vi "update tomo component.vi"(8 "error in (no error)":errorcluster, 11 "Autofocus in":refnum<class "Autofocus.lvclass">) -> (0 "error out":errorcluster, 3 "Autofocus out":refnum<class "Autofocus.lvclass">)   [LabVIEW 2012, in "Autofocus.lvclass"]
uses:
  Autofocus.lvclass
  <vilib>/Distrio/Murmex/Murmex/update_cluster.ctl
  Autofocus.lvclass/Autofocus.ctl
  <vilib>/Distrio/Murmex/Murmex/Murmex.lvclass
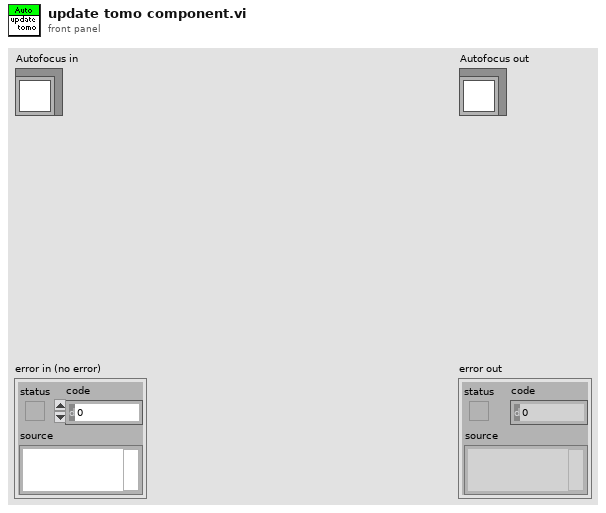
[diagram p1: front panel]
types:
  T1 = typedef "Murmex.lvlib/Murmex.lvclass/update_cluster.ctl" = cluster{"target ID":string, "key chains":string[], "values":variant[]}
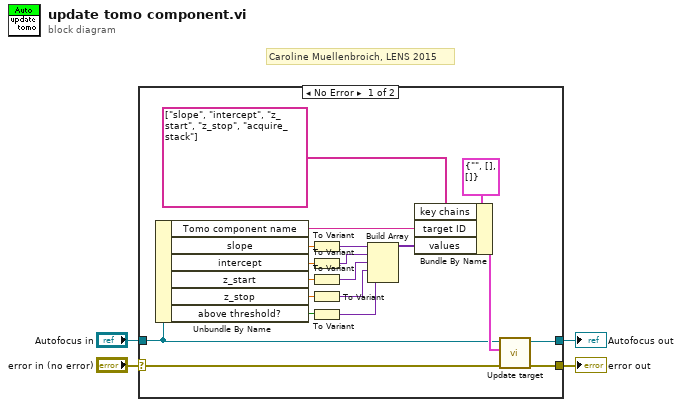
[diagram p0: block diagram]
diagram:
  # "Caroline Muellenbroich, LENS 2015"
  n1 = case shown="No Error" "error in (no error)" {
    selector: "error in (no error)" -> [w17 w25]
    tunnel: [w7 w25] -> w3
    tunnel: [w8 w24] -> w1
    tunnel: "Autofocus in" -> [w16 w24]
    frame No Error {
      n2 = Unbundle By Name(w16) -> ("Tomo component name"=w23:string, "slope"=w12:dbl, "intercept"=w11:dbl, "z_start"=w10:dbl[unit], "z_stop"=w9:dbl[unit], "above threshold?"=w6:bool)
      n3 = To Variant(anything=w12) -> (Variant=w19:variant)
      n4 = To Variant(anything=w11) -> (Variant=w15:variant)
      n5 = To Variant(anything=w10) -> (Variant=w14:variant)
      n6 = To Variant(anything=w9) -> (Variant=w13:variant)
      n7 = To Variant(anything=w6) -> (Variant=w5:variant)
      n8 = Build Array(w19, w15, w14, w13, w5) -> (w20:variant[])
      n9 = Bundle By Name(cluster=T1 {"target ID"="", "key chains"=[], "values"=[]} ("update cluster"), "key chains"=string[] ["slope", "intercept", "z_start", "z_stop", "acquire_stack"], "target ID"=w23, "values"=w20) -> (w21:T1)
      n10 = call <vilib>:"Update target.vi"("error in (no error)"=w17, "update cluster"=w21, "MurmexBase in"=w16) -> ("error out"=w7:errorcluster, "MurmexBase out"=w8:refnum<class "Autofocus.lvclass">)  [unwired: 7 in]
    }
    frame Error {
    }
  }
  "error out" <- w3
  "Autofocus out" <- w1
